vi "getphi.vi"() -> (3 "function return":dbl)   [LabVIEW 2017, in "HapticSTM.lvlib"]
doc: "extern \"C\" __declspec(dllexport) double getphi();"
uses:
  <userlib>/HapticSTM/Feedbackless - Testdata/Zthreshholdtesting 2017 version/Zthreshholdtestingtestytest/HapticSTM.lvlib
  <userlib>/HapticSTM/HapticSTM.dll
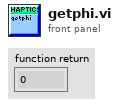
[diagram p1: front panel]
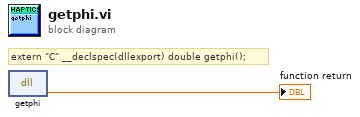
[diagram p0: block diagram]
diagram:
  # "extern \"C\" __declspec(dllexport) double getphi();"
  n1 = dll-call lib="C:/Program Files/National Instruments/LabVIEW 2019/user.lib/HapticSTM/HapticSTM.*" fn="getphi"() -> (→"function return":dbl)  [unwired: 3 in, 2 out]
